vi "Create Output Tag Path.vi"(10 "Channel Name":string, 11 "Group Name":string) -> (3 "Path":string)   [LabVIEW 2020, in "FlexLoggerTagHelpers.lvlib"]
uses:
  FlexLoggerTagHelpers.lvlib
  <vilib>/Skyline/Utilities/NI Skyline Utilities.lvlib
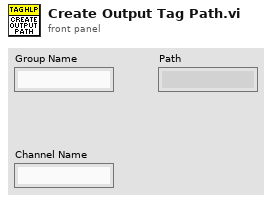
[diagram p1: front panel]
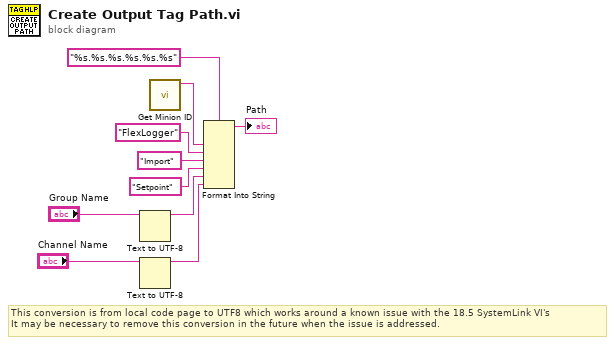
[diagram p0: block diagram]
diagram:
  # "This conversion is from local code page to UTF8 which works around a known issue with the 18.5 SystemLink VI's\nIt may be necessary to remove this conversion in the future when the issue is addressed."
  n1 = Text to UTF-8(11:"Group Name") -> (3:w2:string)  [unwired: 2 in, 1 out]
  n2 = Text to UTF-8(11:"Channel Name") -> (3:w3:string)  [unwired: 2 in, 1 out]
  n3 = call <vilib>:"Get Minion ID.vi"() -> ("minion id"=w7:string)  [unwired: 11 in]
  n4 = Format Into String(format string="%s.%s.%s.%s.%s.%s", w7, "FlexLogger" ("string"), "Import" ("string"), "Setpoint" ("string"), w2, w3) -> (resulting string=→"Path":string)  [unwired: 2 in, 1 out]
